vi "Launcher.vi"(8 "error in (no error)":errorcluster) -> (0 "error out":errorcluster)   [LabVIEW 2016]
doc: "This VI launches the image analyzer application."
uses:
  Controller/Controller/Controller.lvclass
  C:/Program Files (x86)/National Instruments/LabVIEW 2016/vi.lib/ActorFramework/Actor/Actor.lvclass
  <vilib>/ActorFramework/Actor/Actor.lvclass
panel:
  # "Run Me"
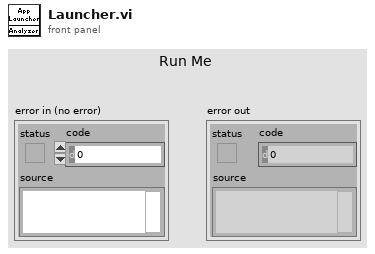
[diagram p1: front panel]
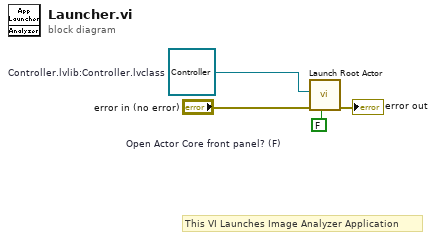
[diagram p0: block diagram]
diagram:
  w1 = FALSE  # Open Actor Core front panel? (F)
  w4 = refnum<class "Controller.lvclass"> refnum  # Controller.lvlib:Controller.lvclass
  # "This VI Launches Image Analyzer Application"
  n1 = call <vilib>:"Launch Root Actor.vi"("Open Actor Core front panel? (F)"=w1, "error in (no error)"="error in (no error)", "Actor"=w4) -> ("error out"=→"error out":errorcluster)  [unwired: 7 in, 1 out]
